vi "PS采集2.vi"   [LabVIEW 2020]
uses:
  Global_Variable/Global.vi
  <userlib>/DAQNavi Polymorphic VI/create/DAQNavi Create Channel(CI-PulseWidth).vi
  <userlib>/DAQNavi Polymorphic VI/read/DAQNavi Read (Counter Pulse Width 1Chan 1Samp).vi
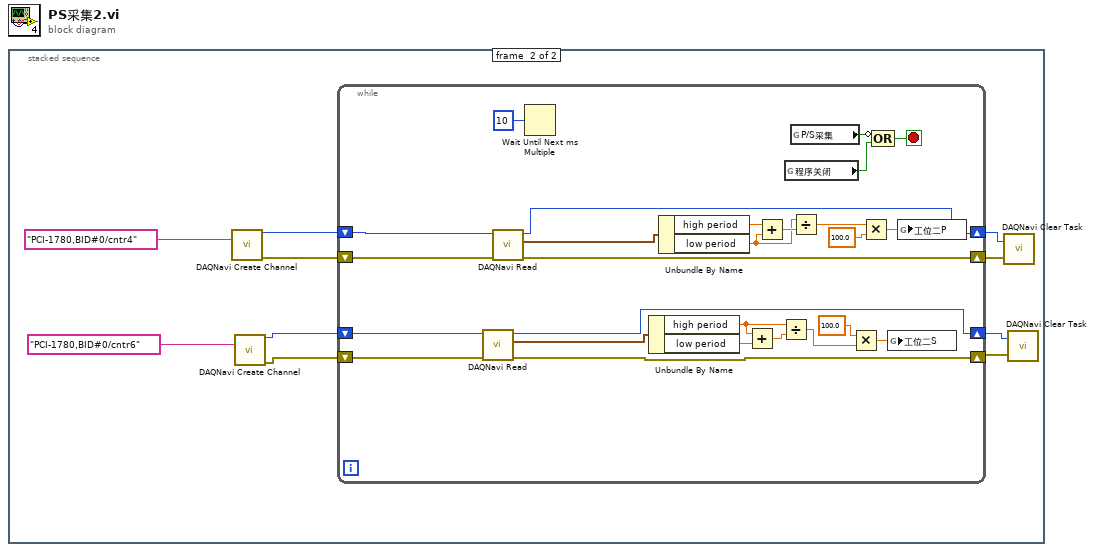
[diagram p0: block diagram]
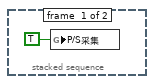
[diagram p2: hidden frame]
diagram:
  n1 = stacked-sequence {
    frame #0 {
      n2 = global write "Global.vi" "P/S采集"(TRUE ("P/S采集")) -> ()
    }
    frame #1 {
      n3 = call-poly <userlib>:"DAQNavi Create Channel.vi"("physical channels"="PCI-1780,BID#0/cntr4") -> ("task out"=w9:i32, "error out"=w8:errorcluster)  [unwired: 13 in]
      n4 = call-poly <userlib>:"DAQNavi Create Channel.vi"("physical channels"="PCI-1780,BID#0/cntr6") -> ("task out"=w5:i32, "error out"=w4:errorcluster)  [unwired: 13 in]
      n5 = while {
        shift-right: [w24] -> w7
        shift-left: w8 -> [w25]
        shift-right: [w13] -> w3
        shift-left: w4 -> [w14]
        shift-right: [w23] -> w6
        shift-left: w9 -> [w26]
        shift-right: [w12] -> w2
        shift-left: w5 -> [w15]
        stop <- w28 stop-if-true
        n6 = call-poly <userlib>:"DAQNavi Read.vi"("error in (no error)"=w14, "task in"=w15) -> ("error out"=w13:errorcluster, "data"=w17:cluster{"high period":dbl, "low period":dbl}, "task out"=w12:i32)  [unwired: 7 in]
        n7 = call-poly <userlib>:"DAQNavi Read.vi"("error in (no error)"=w25, "task in"=w26) -> ("error out"=w24:errorcluster, "data"=w37:cluster{"high period":dbl, "low period":dbl}, "task out"=w23:i32)  [unwired: 7 in]
        n8 = Wait Until Next ms Multiple(millisecond multiple=u32 10 ("毫秒倍数")) -> ()  [unwired: 1 out]
        n9 = Unbundle By Name(w17) -> ("high period"=w21:dbl, "low period"=w19:dbl)
        n10 = Unbundle By Name(w37) -> ("high period"=w36:dbl, "low period"=w34:dbl)
        n11 = Add(x=w21, y=w19) -> (x+y=w18:dbl)
        n12 = Add(x=w36, y=w34) -> (x+y=w35:dbl)
        n13 = Divide(x=w21, y=w18) -> (x/y=w20:dbl)
        n14 = global read "Global.vi" "程序关闭"() -> (w30:bool)
        n15 = global read "Global.vi" "P/S采集"() -> (w29:bool)
        n16 = Divide(x=w34, y=w35) -> (x/y=w33:dbl)
        n17 = Multiply(x=100.0, y=w20) -> (x*y=w22:dbl)
        n18 = Multiply(x=w33, y=100.0) -> (x*y=w31:dbl)
        n19 = Compound Arithmetic op=OR ("复合运算")(invert w29, w30) -> (w28:bool)
        n20 = global write "Global.vi" "工位二S"(w22) -> ()
        n21 = global write "Global.vi" "工位二P"(w31) -> ()
      }
      n22 = call <userlib>:"DAQNavi Clear Task.vi"("error in (no error)"=w7, "task in"=w6) -> ()  [unwired: 1 in, 1 out]
      n23 = call <userlib>:"DAQNavi Clear Task.vi"("error in (no error)"=w3, "task in"=w2) -> ()  [unwired: 1 in, 1 out]
    }
  }
